vi "Initialize Data DVRs.vi"() -> (0 "Data DVRs":T1)   [LabVIEW 2018]
uses:
  Controls/Data Type DVRs.ctl
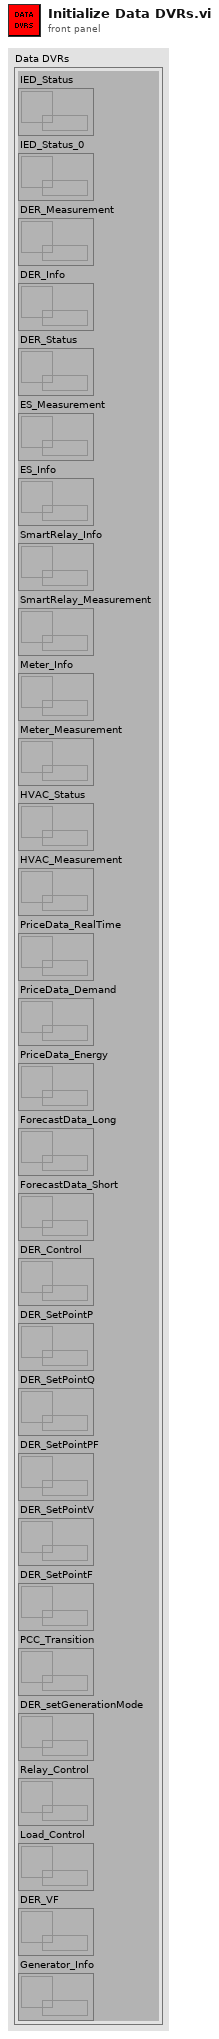
[diagram p1: front panel]
types:
  T1 = typedef "Data Type DVRs.ctl" = cluster{"IED_Status":refnum<data-value>, "IED_Status_0":refnum<data-value>, "DER_Measurement":refnum<data-value>, "DER_Info":refnum<data-value>, "DER_Status":refnum<data-value>, "ES_Measurement":refnum<data-value>, "ES_Info":refnum<data-value>, "SmartRelay_Info":refnum<data-value>, "SmartRelay_Measurement":refnum<data-value>, "Meter_Info":refnum<data-value>, "Meter_Measurement":refnum<data-value>, "HVAC_Status":refnum<data-value>, "HVAC_Measurement":refnum<data-value>, "PriceData_RealTime":refnum<data-value>, "PriceData_Demand":refnum<data-value>, "PriceData_Energy":refnum<data-value>, "ForecastData_Long":refnum<data-value>, "ForecastData_Short":refnum<data-value>, "DER_Control":refnum<data-value>, "DER_SetPointP":refnum<data-value>, "DER_SetPointQ":refnum<data-value>, "DER_SetPointPF":refnum<data-value>, "DER_SetPointV":refnum<data-value>, "DER_SetPointF":refnum<data-value>, "PCC_Transition":refnum<data-value>, "DER_setGenerationMode":refnum<data-value>, "Relay_Control":refnum<data-value>, "Load_Control":refnum<data-value>, "DER_VF":refnum<data-value>, "Generator_Info":refnum<data-value>}
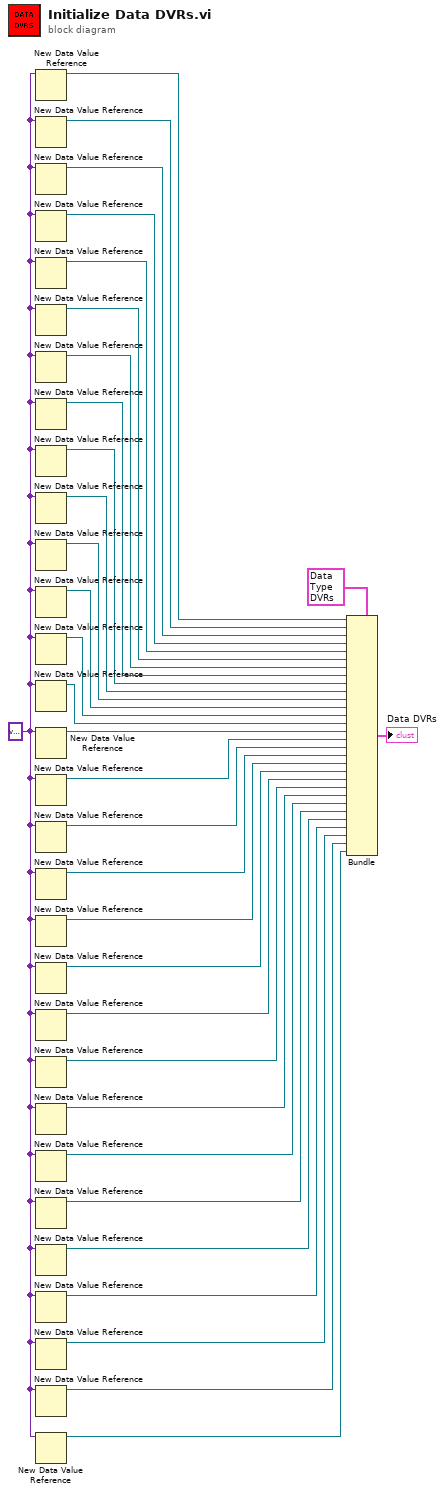
[diagram p0: block diagram]
diagram:
  w4 = variant
  n1 = New Data Value Reference(data value=w4) -> (data value reference=w23:refnum<data-value>)  [unwired: 1 in, 1 out]
  n2 = New Data Value Reference(data value=w4) -> (data value reference=w18:refnum<data-value>)  [unwired: 1 in, 1 out]
  n3 = New Data Value Reference(data value=w4) -> (data value reference=w19:refnum<data-value>)  [unwired: 1 in, 1 out]
  n4 = New Data Value Reference(data value=w4) -> (data value reference=w20:refnum<data-value>)  [unwired: 1 in, 1 out]
  n5 = New Data Value Reference(data value=w4) -> (data value reference=w21:refnum<data-value>)  [unwired: 1 in, 1 out]
  n6 = New Data Value Reference(data value=w4) -> (data value reference=w22:refnum<data-value>)  [unwired: 1 in, 1 out]
  n7 = New Data Value Reference(data value=w4) -> (data value reference=w24:refnum<data-value>)  [unwired: 1 in, 1 out]
  n8 = New Data Value Reference(data value=w4) -> (data value reference=w25:refnum<data-value>)  [unwired: 1 in, 1 out]
  n9 = New Data Value Reference(data value=w4) -> (data value reference=w26:refnum<data-value>)  [unwired: 1 in, 1 out]
  n10 = New Data Value Reference(data value=w4) -> (data value reference=w27:refnum<data-value>)  [unwired: 1 in, 1 out]
  n11 = New Data Value Reference(data value=w4) -> (data value reference=w28:refnum<data-value>)  [unwired: 1 in, 1 out]
  n12 = New Data Value Reference(data value=w4) -> (data value reference=w29:refnum<data-value>)  [unwired: 1 in, 1 out]
  n13 = New Data Value Reference(data value=w4) -> (data value reference=w30:refnum<data-value>)  [unwired: 1 in, 1 out]
  n14 = New Data Value Reference(data value=w4) -> (data value reference=w31:refnum<data-value>)  [unwired: 1 in, 1 out]
  n15 = New Data Value Reference(data value=w4) -> (data value reference=w32:refnum<data-value>)  [unwired: 1 in, 1 out]
  n16 = New Data Value Reference(data value=w4) -> (data value reference=w33:refnum<data-value>)  [unwired: 1 in, 1 out]
  n17 = New Data Value Reference(data value=w4) -> (data value reference=w17:refnum<data-value>)  [unwired: 1 in, 1 out]
  n18 = New Data Value Reference(data value=w4) -> (data value reference=w16:refnum<data-value>)  [unwired: 1 in, 1 out]
  n19 = New Data Value Reference(data value=w4) -> (data value reference=w15:refnum<data-value>)  [unwired: 1 in, 1 out]
  n20 = New Data Value Reference(data value=w4) -> (data value reference=w14:refnum<data-value>)  [unwired: 1 in, 1 out]
  n21 = New Data Value Reference(data value=w4) -> (data value reference=w13:refnum<data-value>)  [unwired: 1 in, 1 out]
  n22 = New Data Value Reference(data value=w4) -> (data value reference=w12:refnum<data-value>)  [unwired: 1 in, 1 out]
  n23 = New Data Value Reference(data value=w4) -> (data value reference=w11:refnum<data-value>)  [unwired: 1 in, 1 out]
  n24 = New Data Value Reference(data value=w4) -> (data value reference=w10:refnum<data-value>)  [unwired: 1 in, 1 out]
  n25 = New Data Value Reference(data value=w4) -> (data value reference=w9:refnum<data-value>)  [unwired: 1 in, 1 out]
  n26 = New Data Value Reference(data value=w4) -> (data value reference=w8:refnum<data-value>)  [unwired: 1 in, 1 out]
  n27 = New Data Value Reference(data value=w4) -> (data value reference=w7:refnum<data-value>)  [unwired: 1 in, 1 out]
  n28 = New Data Value Reference(data value=w4) -> (data value reference=w6:refnum<data-value>)  [unwired: 1 in, 1 out]
  n29 = New Data Value Reference(data value=w4) -> (data value reference=w5:refnum<data-value>)  [unwired: 1 in, 1 out]
  n30 = New Data Value Reference(data value=w4) -> (data value reference=w3:refnum<data-value>)  [unwired: 1 in, 1 out]
  n31 = Bundle(cluster=T1 {"IED_Status"=refnum, "IED_Status_0"=refnum, "DER_Measurement"=refnum, "DER_Info"=refnum, "DER_Status"=refnum, "ES_Measurement"=refnum, "ES_Info"=refnum, "SmartRelay_Info"=refnum, "SmartRelay_Measurement"=refnum, "Meter_Info"=refnum, "Meter_Measurement"=refnum, "HVAC_Status"=refnum, "HVAC_Measurement"=refnum, "PriceData_RealTime"=refnum, "PriceData_Demand"=refnum, "PriceData_Energy"=refnum, "ForecastData_Long"=refnum, "ForecastData_Short"=refnum, "DER_Control"=refnum, "DER_SetPointP"=refnum, "DER_SetPointQ"=refnum, "DER_SetPointPF"=refnum, "DER_SetPointV"=refnum, "DER_SetPointF"=refnum, "PCC_Transition"=refnum, "DER_setGenerationMode"=refnum, "Relay_Control"=refnum, "Load_Control"=refnum, "DER_VF"=refnum, "Generator_Info"=refnum} ("DVR"), "IED_Status"=w23, "IED_Status_0"=w18, "DER_Measurement"=w19, "DER_Info"=w20, "DER_Status"=w21, "ES_Measurement"=w22, "ES_Info"=w24, "SmartRelay_Info"=w25, "SmartRelay_Measurement"=w26, "Meter_Info"=w27, "Meter_Measurement"=w28, "HVAC_Status"=w29, "HVAC_Measurement"=w30, "PriceData_RealTime"=w31, "PriceData_Demand"=w32, "PriceData_Energy"=w33, "ForecastData_Long"=w17, "ForecastData_Short"=w16, "DER_Control"=w15, "DER_SetPointP"=w14, "DER_SetPointQ"=w13, "DER_SetPointPF"=w12, "DER_SetPointV"=w11, "DER_SetPointF"=w10, "PCC_Transition"=w9, "DER_setGenerationMode"=w8, "Relay_Control"=w7, "Load_Control"=w6, "DER_VF"=w5, "Generator_Info"=w3) -> (→"Data DVRs":T1)
